vi "Configuration 1.4 Finalize.vi"(8 "error in (no error)":errorcluster, 10 "file version (1.4)":T2={"major"=1, "minor"=4, "fix"=0, "build"=""}, 11 "configuration 1.4":T1={"plugins"=[{"core"={"name"="", "components"=[], "cycle timing"={"priority"=10000, "decimation"=1, "offset"=0}}, "component settings"=[], "threads"=[{"core"={"processor"=-2, "priority offset"=0}, "component settings"=[], "transfer groups"=[{"core"={"name"="Group", "direction"=enum."Tx", "cycle timing"={"priority"=100, "decimation"=1, "offset"=0}, "timeout behavior"=enum."Increment Late Count", "enable conversion"=FALSE}, "component settings"=[], "transfers"=[{"core"={"name"="Transfer"}, "component settings"=[], "channels"=[{"core"={"name"="Channel", "units"="V", "engine data type"=enum."DBL", "string data type"=enum."DBL", "string offset"=0}, "component settings"=[]}]}]}]}]}]}) -> (0 "error out":errorcluster, 2 "final file version":T2, 3 "configuration json":string)   [LabVIEW 2017, in "DSF Core.lvlib" / "Configuration Session.lvclass"]
uses:
  Configuration Session.lvclass
  Typedefs/DSF Version Info.ctl
  DSF Core.lvlib
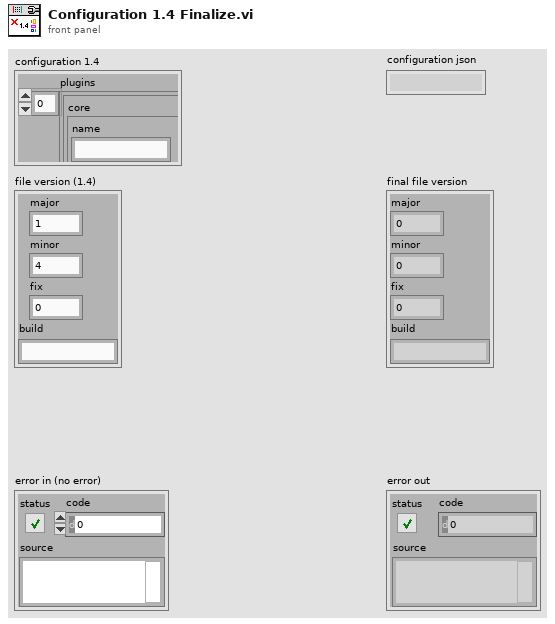
[diagram p1: front panel]
types:
  T1 = cluster{"plugins":cluster{"core":cluster{"name":string, "components":string[], "cycle timing":cluster{"priority":u64, "decimation":u64, "offset":u64}}, "component settings":cluster{"component":string, "values":cluster{"key":string, "value":string}[]}[], "threads":cluster{"core":cluster{"processor":i32, "priority offset":i16}, "component settings":cluster{"component":string, "values":cluster{"key":string, "value":string}[]}[], "transfer groups":cluster{"core":cluster{"name":string, "direction":enum8{"Tx", "Rx"}, "cycle timing":cluster{"priority":u64, "decimation":u64, "offset":u64}, "timeout behavior":enum8{"Increment Late Count", "Throw Error"}, "enable conversion":bool}, "component settings":cluster{"component":string, "values":cluster{"key":string, "value":string}[]}[], "transfers":cluster{"core":cluster{"name":string}, "component settings":cluster{"component":string, "values":cluster{"key":string, "value":string}[]}[], "channels":cluster{"core":cluster{"name":string, "units":string, "engine data type":enum8{"Bool", "SGL", "DBL", "I8", "I16", "I32", "I64", "U8", "U16", "U32", "U64"}, "string data type":enum8{"Bool", "SGL", "DBL", "I8", "I16", "I32", "I64", "U8", "U16", "U32", "U64"}, "string offset":u64}, "component settings":cluster{"component":string, "values":cluster{"key":string, "value":string}[]}[]}[]}[]}[]}[]}[]}
  T2 = typedef "DSF Core.lvlib/DSF Version Info.ctl" = cluster{"major":u32, "minor":u32, "fix":u32, "build":string}
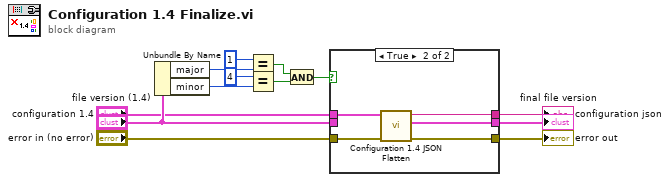
[diagram p0: block diagram]
diagram:
  n1 = Unbundle By Name("file version (1.4)") -> ("major"=w12:u32, "minor"=w13:u32)
  n2 = Equal?(x=u32 1, y=w12) -> (x = y?=w8:bool)
  n3 = Equal?(x=u32 4, y=w13) -> (x = y?=w9:bool)
  n4 = And(x=w8, y=w9) -> (x .and. y?=w7:bool)
  n5 = case shown="True" w7 {
    tunnel: "error in (no error)" -> [w14 w19]
    tunnel: "configuration 1.4" -> [_ w18]
    tunnel: [w14 w17] -> w4
    tunnel: "file version (1.4)" -> [_ _]
    tunnel: [_ w16] -> w5
    tunnel: [_ w15] -> w2
    frame False {
    }
    frame True {
      n6 = call "Configuration 1.4 JSON Flatten.vi"("error in (no error)"=w19, "configuration 1.4"=w18) -> ("error out"=w17:errorcluster, "dsf version"=w15:T2, "dsf configuration json"=w16:string)  [unwired: 7 in]
    }
  }
  "error out" <- w4
  "final file version" <- w2
  "configuration json" <- w5
